vi "parking_ung2rev.vi"() -> ()   [LabVIEW 2012]
uses:
  G_SEN.vi
  G_NAV.vi
  G_VEH.vi
  G_PATH.vi
panel:
  out "M6006":T1={"GPSTime"=22892800.0, "attitude[2]"=-0.6123908, "lcc[0]"=-970.47205, "lcc[1]"=200.52362, "heading_GPS"=-0.6106907} {"GPSTime" format="%#_6f"}
  in  "a":dbl=0.1
  out "parkingpoint":dbl[][](array[numeric])=[[461.5244031818319, -787.8333505670688, 1.0792755610756257], [466.2440748318668, -779.0171892983614, 1.0792755610756257], [467.4239927443755, -776.8131489811844, 1.0792755610756257], [468.60391065688424, -774.6091086640076, 0.48978457392345476], [475.6187081476555, -773.2417442369818, -0.09970641322871643], [485.5690424693232, -774.2371571598643, -0.09970641322871643]]
  out "size":i32=12
  out "sizex":i32=12
  out "sizey":i32=1
  out "xmin":dbl=-1.5
  out "mapzero":dbl[][](array[numeric])
  out "XY Graph":cluster{"Y":dbl[], "Y":dbl[]}[](graph)=[{"Y"=[], "Y"=[]}, {"Y"=[], "Y"=[]}, {"Y"=[], "Y"=[]}, {"Y"=array[1422 elements], "Y"=array[1422 elements]}, {"Y"=[], "Y"=[]}, {"Y"=[0.5023373790116399, 1.0005000639291148, -1.499467549798603, -1.9976302347160777, 0.5023373790116399], "Y"=[3.2753448651924955, -1.6997766347666685, -1.950100285891864, 3.0250212140673, 3.2753448651924955]}]
  out "time":u32
  out "box":dbl[][](array[numeric])
  out "lane":dbl[][](array[numeric])
  out "obs":dbl[][](array[numeric])
  out "y_min":dbl=-2.25
  out "tic":u32=336134883
  out "sensor_lane":dbl[][](array[numeric])
  out "sensor_obs":dbl[][](array[numeric])
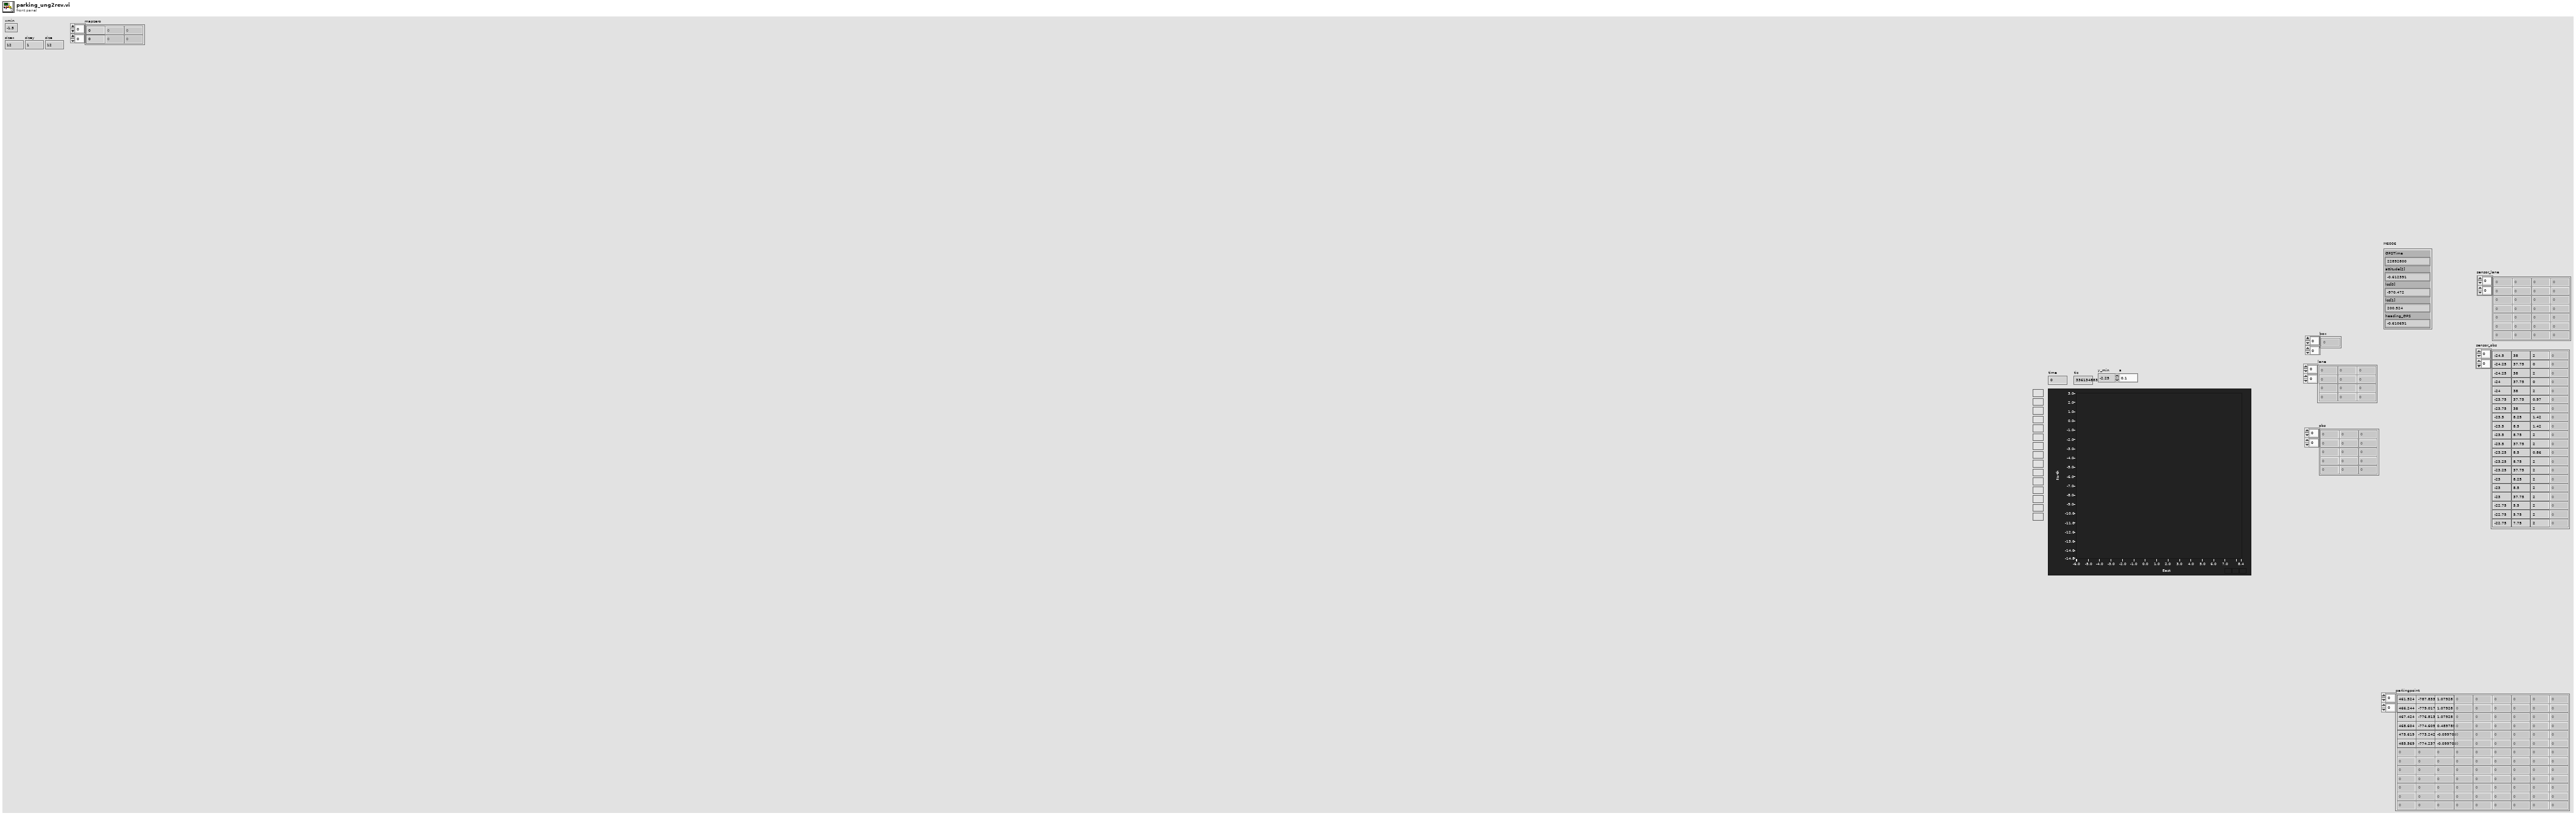
[diagram p1: front panel]
types:
  T1 = cluster{"GPSTime":dbl, "attitude[2]":sgl, "lcc[0]":sgl, "lcc[1]":sgl, "heading_GPS":sgl}
  T2 = cluster{"GPSTime":dbl, "attitude[2]":dbl, "lcc[0]":dbl, "lcc[1]":dbl, "heading_GPS":dbl}
  T3 = cluster{"idx":i32, "x":dbl, "y":dbl, "h":dbl, "x_path":dbl}
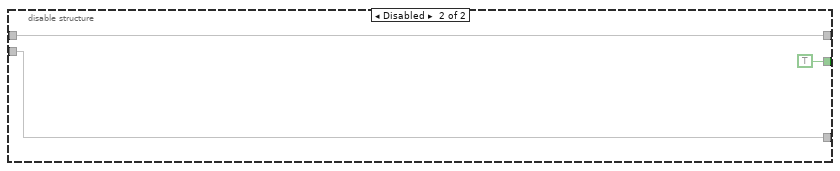
[diagram p3: hidden frame]
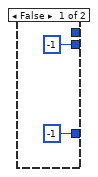
[diagram p6: hidden frame]
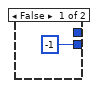
[diagram p7: hidden frame]
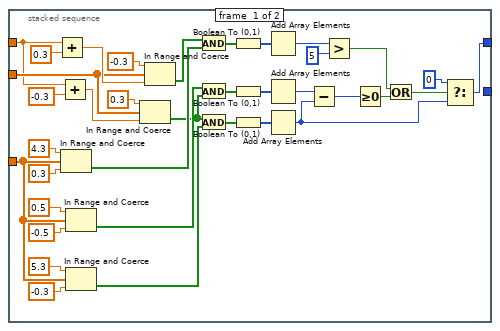
[diagram p8: hidden frame]
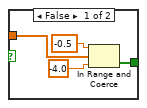
[diagram p10: hidden frame]
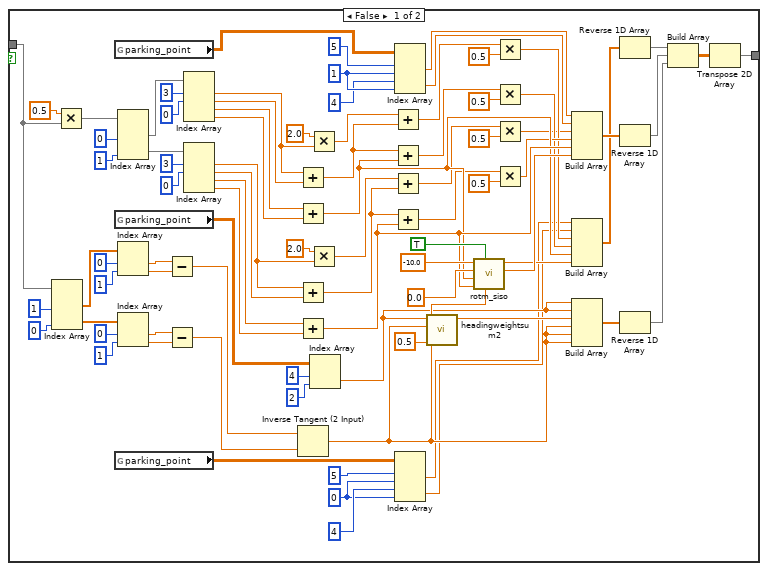
[diagram p13: hidden frame]
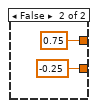
[diagram p16: hidden frame]
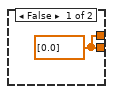
[diagram p17: hidden frame]
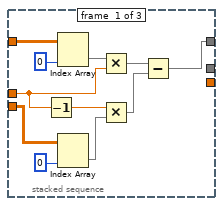
[diagram p18: hidden frame]
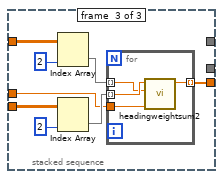
[diagram p19: hidden frame]
diagram:
  n1 = flat-sequence {
    tunnel: [w865] -> w2
    tunnel: [w864] -> w1
    tunnel: w2 -> [w878]
    tunnel: w1 -> [w877]
    frame #0 {
      n2 = disable-structure shown="Disabled" {
        disable-tunnel: [w10 _] -> w7
        frame Disabled {
          n3 = local read "sensor_obs"() -> (w10:dbl[][])
        }
        frame Enabled {
        }
      }
      "obs" <- w7
      n4 = Tick Count (ms)() -> (millisecond timer value=→"tic":u32)
      n5 = global read "G_SEN.vi" "sensor_lane"() -> (w6:dbl[][])
      n6 = global read "G_SEN.vi" "sensor_obs"() -> (→"sensor_obs":dbl[][])
      n7 = global read "G_SEN.vi" "sensor_etc"() -> (w5:dbl[][])
      n8 = global read "G_NAV.vi" "M6006"() -> (→"M6006":T2)
      n9 = Build Array (concatenate)(w5, w6) -> (→"sensor_lane":dbl[][])
    }
    frame #1 {
      n10 = local read "sensor_lane"() -> (w17:dbl[][])
      n11 = Index Array(array=w17, index (col) #1=0 ("disabled index (col)")) -> (element #1=w15:dbl[], element #2=w14:dbl[])  [unwired: 3 in]
      n12 = disable-structure shown="Enabled" {
        disable-tunnel: w15 -> [w31 w57]
        disable-tunnel: w14 -> [w30 w56]
        disable-tunnel: [w21 w56] -> w13
        disable-tunnel: [w22 w57] -> w12
        disable-tunnel: [w26 TRUE] -> w11
        frame Enabled {
          n13 = local read "M6006"() -> (w47:T1)
          n14 = Unbundle By Name(w47) -> ("lcc[1]"=w44:sgl, "lcc[0]"=w45:sgl, "attitude[2]"=w46:sgl)
          n15 = global read "G_VEH.vi" "xparking"() -> (w50:T3)
          n16 = Negate(x=w46) -> (-x=w43:sgl)
          n17 = Unbundle By Name(w50) -> ("x"=w49:dbl, "y"=w48:dbl)
          n18 = call "rotm_siso.vi"("angle[rad]"=w43, "y0"=w45, "x0"=w44, "y"=w48, "x"=w49) -> ("y'"=w41:dbl, "x'"=w42:dbl)  [unwired: 5 in]
          n19 = Subtract(x=w31, y=w42) -> (x-y=w39:dbl[])
          n20 = Subtract(x=w30, y=w41) -> (x-y=w40:dbl[])
          n21 = Square(x=w39) -> (x^2=w38:dbl[])
          n22 = Square(x=w40) -> (x^2=w37:dbl[])
          n23 = Add(x=w38, y=w37) -> (x+y=w36:dbl[])
          n24 = Square Root(x=w36) -> (sqrt(x)=w35:dbl[])
          n25 = Less Or Equal?(x=w35, y=3.0) -> (x <= y?=w33:bool[])
          n26 = Boolean To (0,1)(Boolean=w33) -> (0, 1=w32:i16[])
          n27 = Build Cluster Array(w32, w31, w30) -> (w29:cluster{i16, "element":dbl, "element":dbl}[])
          n28 = Sort 1D Array(array=w29) -> (sorted array=w28:cluster{i16, "element":dbl, "element":dbl}[])
          n29 = for {
            tunnel: w28 -> [w54] mode=indexing
            tunnel: [w53] -> w25 mode=indexing
            tunnel: [w52] -> w24 mode=indexing
            tunnel: [w51] -> w23 mode=indexing
            n30 = Unbundle(w54) -> (w51:i16, "element"=w53:dbl, "element"=w52:dbl)
          }
          n31 = Add Array Elements(numeric array=w23) -> (sum=w19:i16)
          n32 = Array Max & Min(array=w23) -> (max value=w27:i16, max index (indices)=w20:i32)  [unwired: 2 out]
          n33 = Not Equal To 0?(x=w27) -> (x != 0?=w26:bool)
          n34 = Array Subset(array=w25, index=w20, length=w19) -> (w22:dbl[])
          n35 = Array Subset(array=w24, index=w20, length=w19) -> (w21:dbl[])
        }
        frame Disabled {
        }
      }
      n36 = case shown="True" w11 {
        tunnel: w13 -> [_ w58]
        tunnel: w12 -> [_ w60]
        tunnel: [_ w66] -> w18
        frame False {
        }
        frame True {
          n37 = Array Max & Min(array=w60) -> (max value=w65:dbl, min value=w64:dbl)  [unwired: 2 out]
          n38 = Array Max & Min(array=w58) -> (max value=w63:dbl, min value=w62:dbl)  [unwired: 2 out]
          n39 = flat-sequence {
            tunnel: w65 -> [w79]
            tunnel: w64 -> [w78]
            tunnel: w63 -> [w77]
            tunnel: w62 -> [w76]
            tunnel: [w69] -> w61
            tunnel: w60 -> [w69]
            tunnel: [w68] -> w59
            tunnel: w58 -> [w68]
            tunnel: [w117] -> w67
            tunnel: w61 -> [w106]
            tunnel: w59 -> [w105]
            tunnel: w67 -> [w148]
            tunnel: [w147] -> w66
            frame #0 {
              n40 = flat-sequence {
                tunnel: w79 -> [w83]
                tunnel: w78 -> [w82]
                tunnel: w77 -> [_]
                tunnel: w76 -> [w81]
                tunnel: [w83] -> w75
                tunnel: [w82] -> w74
                tunnel: [0.0] -> w73
                tunnel: [w81] -> w72
                tunnel: w75 -> [w100]
                tunnel: w74 -> [w99]
                tunnel: w73 -> [w94]
                tunnel: w72 -> [w93]
                tunnel: [w91] -> w71
                tunnel: [w90] -> w70
                tunnel: w71 -> [w103]
                tunnel: w70 -> [w102]
                frame #0 {
                  "y_min" <- w81
                  "xmin" <- w82
                }
                frame #1 {
                  n41 = Subtract(x=w100, y=w99) -> (x-y=w98:dbl)
                  n42 = Subtract(x=w94, y=w93) -> (x-y=w95:dbl)
                  n43 = Multiply(x=w98, y=4.0) -> (x*y=w89:dbl)
                  n44 = Multiply(x=w95, y=4.0) -> (x*y=w88:dbl)
                  n45 = Round Toward +Infinity(x=w89) -> (ceil(x): smallest int >= x=w84:dbl)
                  n46 = Round Toward +Infinity(x=w88) -> (ceil(x): smallest int >= x=w87:dbl)
                  n47 = Increment(x=w84) -> (x+1=w85:dbl)
                  n48 = Increment(x=w87) -> (x+1=w86:dbl)
                  n49 = To Long Integer(number=w85) -> (32bit integer=w91:i32)
                  "sizex" <- w91
                  n50 = To Long Integer(number=w86) -> (32bit integer=w90:i32)
                  "sizey" <- w90
                  n51 = Multiply(x=w91, y=w90) -> (x*y=→"size":i32)
                }
                frame #2 {
                  n52 = Initialize Array(0.0, w103, w102) -> (→"mapzero":dbl[][])
                }
              }
            }
            frame #1 {
              n53 = local read "y_min"() -> (w111:dbl)
              n54 = local read "xmin"() -> (w108:dbl)
              n55 = local read "mapzero"() -> (w107:dbl[][])
              n56 = Subtract(x=w106, y=w108) -> (x-y=w116:dbl[])
              n57 = Subtract(x=w105, y=w111) -> (x-y=w110:dbl[])
              n58 = Multiply(x=w116, y=4.0) -> (x*y=w114:dbl[])
              n59 = Multiply(x=4.0, y=w110) -> (x*y=w115:dbl[])
              n60 = To Long Integer(number=w114) -> (32bit integer=w113:i32[])
              n61 = To Long Integer(number=w115) -> (32bit integer=w112:i32[])
              n62 = for {
                tunnel: w113 -> [w123] mode=indexing
                shift-right: [w122] -> w117
                shift-left: w107 -> [w120]
                tunnel: w112 -> [w121] mode=indexing
                n63 = Replace Array Subset(array=w120, new element=1.0 ("new element/subarray"), index (row)=w123, index (col)=w121) -> (w122:dbl[][])
              }
            }
            frame #2 {
              n64 = local read "sizey"() -> (w138:i32)
              n65 = local read "sizex"() -> (w143:i32)
              n66 = local read "size"() -> (w124:i32)
              n67 = for {
                N: w138 -> [_]
                tunnel: [w168] -> w137 mode=indexing
                i -> [w168]
              }
              n68 = Reshape Array(w148, w124) -> (w144:dbl[])
              n69 = for {
                N: w143 -> [_]
                tunnel: [w169] -> w142 mode=concatenating
                i -> [w171]
                n70 = local read "sizey"() -> (w170:i32)
                n71 = Initialize Array(w171, w170) -> (w169:i32[])
              }
              n72 = Not Equal To 0?(x=w144) -> (x != 0?=w126:bool[])
              n73 = Boolean To (0,1)(Boolean=w126) -> (0, 1=w131:i16[])
              n74 = Add Array Elements(numeric array=w131) -> (sum=w129:i16)
              n75 = Multiply(x=w137, y=0.25) -> (x*y=w134:dbl[])
              n76 = local read "y_min"() -> (w135:dbl)
              n77 = Multiply(x=w142, y=0.25) -> (x*y=w139:dbl[])
              n78 = local read "xmin"() -> (w140:dbl)
              n79 = Add(x=w134, y=w135) -> (x+y=w132:dbl[])
              n80 = local read "sizex"() -> (w133:i32)
              n81 = Add(x=w139, y=w140) -> (x+y=w146:dbl[])
              n82 = for {
                N: w133 -> [_]
                tunnel: w132 -> [w167]
                tunnel: [w167] -> w145 mode=concatenating
              }
              n83 = Initialize Array(0.0 ("element"), w129, 3 ("dimension size")) -> (w127:dbl[][])
              n84 = for {
                tunnel: w145 -> [w156] mode=indexing
                tunnel: w146 -> [w155] mode=indexing
                tunnel: w144 -> [w152] mode=indexing
                shift-right: [w153] -> w147
                shift-left: w127 -> [w154]
                tunnel: w126 -> [w151] mode=indexing
                shift-right: [w149] -> _
                shift-left: 0 -> [w150]
                n85 = case shown="True" w151 {
                  tunnel: w156 -> [_ w165]
                  tunnel: w155 -> [_ w166]
                  tunnel: w152 -> [_ w164]
                  tunnel: w154 -> [w158 w163]
                  tunnel: [w158 w162] -> w153
                  tunnel: w150 -> [w157 w160]
                  tunnel: [w157 w159] -> w149
                  frame False {
                  }
                  frame True {
                    n86 = Build Array(w166, w165, w164) -> (w161:dbl[])
                    n87 = Increment(x=w160) -> (x+1=w159:i32)
                    n88 = Replace Array Subset(array=w163, new element=w161, index (row)=w160) -> (w162:dbl[][])  [unwired: 1 in]
                  }
                }
              }
            }
          }
        }
      }
      "lane" <- w18
    }
    frame #2 {
      n89 = flat-sequence {
        tunnel: [w173] -> w172
        frame #0 {
          n90 = flat-sequence {
            tunnel: [w181] -> w176
            tunnel: [w179] -> w175
            tunnel: [w180] -> w174
            tunnel: w176 -> [w318]
            tunnel: w175 -> [w324]
            tunnel: w174 -> [w319]
            tunnel: [w316] -> w173
            frame #0 {
              n91 = local read "lane"() -> (w183:dbl[][])
              n92 = Index Array(array=w183, index (col) #1=1 ("disabled index (col)"), index (col) #2=0 ("index (col)")) -> (element #1=w178:dbl[], element #2=w177:dbl[])  [unwired: 2 in]
              n93 = for {
                tunnel: w177 -> [w192]
                tunnel: w178 -> [w193]
                tunnel: [w198] -> w181 mode=indexing
                tunnel: [w197] -> w180 mode=indexing
                tunnel: [w196] -> w179 mode=indexing
                tunnel: w178 -> [w191] mode=indexing
                tunnel: w177 -> [w190] mode=indexing
                n94 = Subtract(x=w193, y=w191) -> (x-y=w202:dbl[])
                n95 = Subtract(x=w192, y=w190) -> (x-y=w201:dbl[])
                n96 = global read "G_PATH.vi" "parking_width"() -> (w185:dbl)
                n97 = Square(x=w202) -> (x^2=w205:dbl[])
                n98 = Square(x=w201) -> (x^2=w204:dbl[])
                n99 = Inverse Tangent (2 Input)(1:w201, 2:w202) -> (0:w195:dbl[])
                n100 = Add(x=w205, y=w204) -> (x+y=w200:dbl[])
                n101 = Square Root(x=w200) -> (sqrt(x)=w199:dbl[])
                n102 = Add(x=0.6, y=w185) -> (x+y=w186:dbl)
                n103 = Subtract(x=w185, y=0.6) -> (x-y=w188:dbl)
                n104 = In Range and Coerce(upper limit=w186, x=w199, lower limit=w188) -> (In Range?=w194:bool[])  [unwired: 1 out]
                n105 = Or Array Elements(Boolean array=w194) -> (logical OR=w203:bool)
                n106 = case shown="True" w203 {
                  tunnel: w194 -> [_ w220]
                  tunnel: w202 -> [_ w219]
                  tunnel: w201 -> [_ w218]
                  tunnel: w195 -> [_ w217]
                  tunnel: w199 -> [_ w210]
                  tunnel: [_ w212] -> w198
                  tunnel: [-1 ("element") w216] -> w197
                  tunnel: [-1 ("element") w213] -> w196
                  frame False {
                  }
                  frame True {
                    n107 = Negate(x=w210) -> (-x=w209:dbl[])
                    n108 = for {
                      tunnel: w220 -> [w228] mode=indexing
                      tunnel: w219 -> [w227]
                      tunnel: w218 -> [w226]
                      tunnel: w217 -> [w225] mode=indexing
                      tunnel: w209 -> [w224] mode=indexing
                      tunnel: [w223] -> w215 mode=indexing
                      tunnel: [w222] -> w214 mode=indexing
                      tunnel: [w221] -> w208 mode=indexing
                      i -> [w222]
                      n109 = case shown="True" w228 {
                        tunnel: w227 -> [_ w242]
                        tunnel: w226 -> [_ w241]
                        tunnel: w225 -> [_ w239]
                        tunnel: w224 -> [_ w235]
                        tunnel: [-1 w230] -> w223
                        tunnel: [_ w231] -> w221
                        frame False {
                        }
                        frame True {
                          w240 = 0.0 ("y0")
                          n110 = call "rotm_mimo.vi"("angle[rad]"=w239, "y0"=w240, "x0"=w240, "y"=w242, "x"=w241) -> ("Y"=w237:dbl[], "X"=w238:dbl[])  [unwired: 3 in, 2 out]
                          n111 = Negate(x=w238) -> (-x=w236:dbl[])
                          n112 = stacked-sequence {
                            tunnel: w237 -> [w256 w293]
                            tunnel: w236 -> [w261 w297]
                            tunnel: w235 -> [w260 w296]
                            tunnel: [w259 _] -> w234
                            tunnel: [_ w283] -> w233
                            frame #0 {
                              n113 = Add(x=w260, y=0.3) -> (x+y=w266:dbl)
                              n114 = Add(x=w260, y=-0.3) -> (x+y=w274:dbl)
                              n115 = In Range and Coerce(upper limit=4.3, x=w256, lower limit=0.3) -> (In Range?=w268:bool[])  [unwired: 1 out]
                              n116 = In Range and Coerce(upper limit=0.5, x=w256, lower limit=-0.5) -> (In Range?=w255:bool[])  [unwired: 1 out]
                              n117 = In Range and Coerce(upper limit=5.3, x=w256, lower limit=-0.3) -> (In Range?=w273:bool[])  [unwired: 1 out]
                              n118 = In Range and Coerce(upper limit=0.3, x=w261, lower limit=w274) -> (In Range?=w254:bool[])  [unwired: 1 out]
                              n119 = In Range and Coerce(upper limit=-0.3, x=w261, lower limit=w266) -> (In Range?=w267:bool[])  [unwired: 1 out]
                              n120 = And(x=w267, y=w268) -> (x .and. y?=w269:bool[])
                              n121 = And(x=w255, y=w254) -> (x .and. y?=w252:bool[])
                              n122 = And(x=w254, y=w273) -> (x .and. y?=w272:bool[])
                              n123 = Boolean To (0,1)(Boolean=w269) -> (0, 1=w270:i16[])
                              n124 = Boolean To (0,1)(Boolean=w252) -> (0, 1=w253:i16[])
                              n125 = Boolean To (0,1)(Boolean=w272) -> (0, 1=w271:i16[])
                              n126 = Add Array Elements(numeric array=w270) -> (sum=w246:i16)
                              n127 = Add Array Elements(numeric array=w253) -> (sum=w251:i16)
                              n128 = Add Array Elements(numeric array=w271) -> (sum=w244:i16)
                              n129 = Subtract(x=w251, y=w244) -> (x-y=w250:i16)
                              n130 = Greater?(x=w246, y=i16 5) -> (0:w249:bool)
                              n131 = Greater Or Equal To 0?(x=w250) -> (x >= 0?=w248:bool)
                              n132 = Or(x=w249, y=w248) -> (x .or. y?=w247:bool)
                              n133 = Select(t=i16 0, s=w247, f=w244) -> (s? t:f=w259:i16)
                            }
                            frame #1 {
                              n134 = Add(x=w296, y=0.3) -> (x+y=w302:dbl)
                              n135 = Add(x=w296, y=-0.3) -> (x+y=w310:dbl)
                              n136 = In Range and Coerce(upper limit=-0.3, x=w293, lower limit=-4.3) -> (In Range?=w304:bool[])  [unwired: 1 out]
                              n137 = In Range and Coerce(upper limit=0.5, x=w293, lower limit=-0.5) -> (In Range?=w292:bool[])  [unwired: 1 out]
                              n138 = In Range and Coerce(upper limit=0.3, x=w293, lower limit=-5.3) -> (In Range?=w309:bool[])  [unwired: 1 out]
                              n139 = In Range and Coerce(upper limit=0.3, x=w297, lower limit=w310) -> (In Range?=w291:bool[])  [unwired: 1 out]
                              n140 = In Range and Coerce(upper limit=-0.3, x=w297, lower limit=w302) -> (In Range?=w303:bool[])  [unwired: 1 out]
                              n141 = And(x=w303, y=w304) -> (x .and. y?=w305:bool[])
                              n142 = And(x=w292, y=w291) -> (x .and. y?=w289:bool[])
                              n143 = And(x=w291, y=w309) -> (x .and. y?=w308:bool[])
                              n144 = Boolean To (0,1)(Boolean=w305) -> (0, 1=w306:i16[])
                              n145 = Boolean To (0,1)(Boolean=w289) -> (0, 1=w290:i16[])
                              n146 = Boolean To (0,1)(Boolean=w308) -> (0, 1=w307:i16[])
                              n147 = Add Array Elements(numeric array=w306) -> (sum=w282:i16)
                              n148 = Add Array Elements(numeric array=w290) -> (sum=w288:i16)
                              n149 = Add Array Elements(numeric array=w307) -> (sum=w280:i16)
                              n150 = Subtract(x=w288, y=w280) -> (x-y=w287:i16)
                              n151 = Greater?(x=w282, y=i16 5) -> (0:w286:bool)
                              n152 = Greater Or Equal To 0?(x=w287) -> (x >= 0?=w285:bool)
                              n153 = Or(x=w286, y=w285) -> (x .or. y?=w284:bool)
                              n154 = Select(t=i16 0, s=w284, f=w280) -> (s? t:f=w283:i16)
                            }
                          }
                          n155 = Build Array(w234, w233) -> (w232:i16[])
                          n156 = Array Max & Min(array=w232) -> (max value=w231:i16, max index (indices)=w230:i32)  [unwired: 2 out]
                        }
                      }
                    }
                    n157 = Array Max & Min(array=w208) -> (max value=w212:i16, max index (indices)=w211:i32)  [unwired: 2 out]
                    n158 = Index Array(array=w214, index=w211) -> (element=w213:i32)
                    n159 = Index Array(array=w215, index=w211) -> (element=w216:i32)
                  }
                }
              }
            }
            frame #1 {
              n160 = Array Max & Min(array=w318) -> (max value=w320:i16, max index (indices)=w315:i32)  [unwired: 2 out]
              n161 = Index Array(array=w324, index=w315) -> (element=w321:i32)
              n162 = Index Array(array=w319, index=w315) -> (element=w322:i32)
              n163 = Greater Or Equal?(x=w320, y=i16 4) -> (x >= y?=w317:bool)
              n164 = case shown="True" w317 {
                tunnel: w321 -> [_ w364]
                tunnel: w322 -> [_ w342]
                tunnel: [_ w341] -> w316
                tunnel: w315 -> [_ w325]
                frame False {
                }
                frame True {
                  w347 = 0.0 ("element")
                  w344 = dbl[] [0.0, 5.0, 5.0, 0.0]
                  n165 = local read "lane"() -> (w365:dbl[][])
                  n166 = Negate(x=w344) -> (-x=w343:dbl[])
                  n167 = Index Array(array=w365, index (row) #1=w364, index (row) #2=w325) -> (element #1=w363:dbl[], element #2=w357:dbl[])  [unwired: 2 in]
                  n168 = Equal To 0?(x=w342) -> (x = 0?=w326:bool)
                  n169 = Subtract(x=w363, y=w357) -> (x-y=w351:dbl[])
                  n170 = Select(t=w344, s=w326, f=w343) -> (s? t:f=w345:dbl[])
                  n171 = Square(x=w351) -> (x^2=w350:dbl[])
                  n172 = Index Array(array=w351, index #1=1 ("index"), index #2=0 ("index")) -> (element #1=w360:dbl, element #2=w359:dbl)
                  n173 = Add Array Elements(numeric array=w350) -> (sum=w349:dbl)
                  n174 = Inverse Tangent (2 Input)(1:w359, 2:w360) -> (0:w353:dbl)
                  n175 = Square Root(x=w349) -> (sqrt(x)=w348:dbl)
                  n176 = call "headingoperater.vi"("h1"=w353, "h2"=1.5707963267948966) -> ("h2+h1"=w331:dbl)  [unwired: 8 in, 1 out]
                  n177 = Negate(x=w348) -> (-x=w327:dbl)
                  n178 = Index Array(array=w357, index #1=0 ("index")) -> (element #1=w333:dbl, element #2=w332:dbl)  [unwired: 1 in]
                  n179 = flat-sequence {
                    tunnel: [w371] -> w330
                    tunnel: w333 -> [w370]
                    tunnel: w332 -> [w369]
                    tunnel: w331 -> [w368]
                    tunnel: w327 -> [w367]
                    tunnel: w326 -> [w366]
                    frame #0 {
                      n180 = disable-structure shown="Enabled" {
                        disable-tunnel: [w379 _] -> w371
                        disable-tunnel: w370 -> [w378 _]
                        disable-tunnel: w369 -> [w377 _]
                        disable-tunnel: w368 -> [w376 _]
                        disable-tunnel: w367 -> [w375 _]
                        disable-tunnel: w366 -> [w374 _]
                        frame Enabled {
                          n181 = local read "sensor_obs"() -> (w391:dbl[][])
                          n182 = Index Array(array=w391, index (col) #1=0 ("disabled index (col)"), index (col) #2=1 ("index (col)")) -> (element #1=w388:dbl[], element #2=w387:dbl[])  [unwired: 2 in]
                          n183 = call "rotm_mimo.vi"("angle[rad]"=w376, "reverse"=FALSE, "y0"=w377, "x0"=w378, "y"=w387, "x"=w388) -> ("Y"=w383:dbl[], "X"=w385:dbl[])  [unwired: 2 in, 2 out]
                          n184 = Add(x=0.2, y=w375) -> (x+y=w381:dbl)
                          n185 = case shown="True" w374 {
                            tunnel: w385 -> [w394 w399]
                            tunnel: [w392 w396] -> w373
                            frame False {
                              n186 = In Range and Coerce(upper limit=-0.5, x=w394, lower limit=-4.0) -> (In Range?=w392:bool[])  [unwired: 1 out]
                            }
                            frame True {
                              n187 = In Range and Coerce(upper limit=4.0, x=w399, lower limit=0.5) -> (In Range?=w396:bool[])  [unwired: 1 out]
                            }
                          }
                          n188 = In Range and Coerce(upper limit=-0.2, x=w383, lower limit=w381) -> (In Range?=w372:bool[])  [unwired: 1 out]
                          n189 = And(x=w372, y=w373) -> (x .and. y?=w380:bool[])
                          n190 = Or Array Elements(Boolean array=w380) -> (logical OR=w379:bool)
                        }
                        frame Disabled {
                        }
                      }
                    }
                  }
                  n191 = Build Array(w347, w347, w327, w327) -> (w346:dbl[])
                  n192 = call "rotm_mimo.vi"("angle[rad]"=w331, "reverse"=TRUE, "y0"=w332, "x0"=w333, "y"=w346, "x"=w345) -> ("Y"=w355:dbl[], "X"=w338:dbl[])  [unwired: 2 in, 2 out]
                  n193 = Add Array Elements(numeric array=w338) -> (sum=w337:dbl)
                  n194 = Build Array(w338, w355) -> (w354:dbl[][])
                  n195 = Transpose 2D Array(2D array=w354) -> (transposed array=w340:dbl[][])
                  n196 = Multiply(x=0.25, y=w337) -> (x*y=w335:dbl)
                  n197 = Greater?(x=w335, y=7.0) -> (0:w329:bool)
                  n198 = Or(x=w330, y=w329) -> (x .or. y?=w328:bool)
                  n199 = Select(t=dbl[][] [], s=w328, f=w340) -> (s? t:f=w341:dbl[][])
                }
              }
            }
          }
        }
      }
      "box" <- w172
    }
    frame #3 {
      n200 = local read "box"() -> (w401:dbl[][])
      n201 = Empty Array?(array=w401) -> (empty?=w400:bool)
      n202 = case shown="False" w400 {
        frame False {
          n203 = flat-sequence {
            tunnel: [w406] -> w402
            tunnel: w402 -> [w488]
            frame #0 {
              n204 = local read "M6006"() -> (w444:T1)
              n205 = local read "box"() -> (w409:dbl[][])
              n206 = Unbundle By Name(w444) -> ("lcc[1]"=w440:sgl, "lcc[0]"=w439:sgl, "attitude[2]"=w443:sgl)
              n207 = Array Subset(array=w409, length (row)=4 ("length")) -> (w408:dbl[][])  [unwired: 3 in]
              n208 = Negate(x=w443) -> (-x=w442:sgl)
              n209 = Index Array(array=w408, index (col) #1=0 ("disabled index (col)")) -> (element #1=w446:dbl[], element #2=w445:dbl[])  [unwired: 3 in]
              n210 = call "rotm_mimo.vi"("angle[rad]"=w442, "reverse"=TRUE, "y0"=w439, "x0"=w440, "y"=w445, "x"=w446) -> ("Y"=w431:dbl[], "X"=w433:dbl[])  [unwired: 2 in, 2 out]
              n211 = Subtract(x=w433, y=w440) -> (x-y=w437:dbl[])
              n212 = Subtract(x=w431, y=w439) -> (x-y=w438:dbl[])
              n213 = Square(x=w437) -> (x^2=w436:dbl[])
              n214 = Square(x=w438) -> (x^2=w435:dbl[])
              n215 = Add(x=w436, y=w435) -> (x+y=w434:dbl[])
              n216 = Array Max & Min(array=w434) -> (min index (indices)=w432:i32)  [unwired: 3 out]
              n217 = Delete From Array(array=w433, index=w432) -> (deleted portion=w419:dbl, array with subset deleted=w423:dbl[])  [unwired: 1 in]
              n218 = Delete From Array(array=w431, index=w432) -> (deleted portion=w403:dbl, array with subset deleted=w415:dbl[])  [unwired: 1 in]
              n219 = Subtract(x=w423, y=w419) -> (x-y=w427:dbl[])
              n220 = Subtract(x=w415, y=w403) -> (x-y=w426:dbl[])
              n221 = Square(x=w427) -> (x^2=w428:dbl[])
              n222 = Square(x=w426) -> (x^2=w429:dbl[])
              n223 = Add(x=w428, y=w429) -> (x+y=w430:dbl[])
              n224 = Array Max & Min(array=w430) -> (max index (indices)=w413:i32, min index (indices)=w412:i32)  [unwired: 2 out]
              n225 = Add(x=w413, y=w412) -> (x+y=w425:i32)
              n226 = Subtract(x=3, y=w425) -> (x-y=w414:i32)
              n227 = Index Array(array=w423, index #1=w414, index #2=w413, index #3=w412) -> (element #1=w422:dbl, element #2=w421:dbl, element #3=w420:dbl)
              n228 = Index Array(array=w415, index #1=w414, index #2=w413, index #3=w412) -> (element #1=w416:dbl, element #2=w417:dbl, element #3=w418:dbl)
              n229 = Build Array(w419, w422, w421, w420) -> (w411:dbl[])
              n230 = Build Array(w403, w416, w417, w418) -> (w410:dbl[])
              n231 = flat-sequence {
                tunnel: w410 -> [w448]
                tunnel: w411 -> [w451]
                tunnel: [w450] -> w405
                tunnel: [w449] -> w404
                tunnel: [w483] -> w406
                tunnel: w405 -> [w486]
                tunnel: w404 -> [w485]
                frame #0 {
                  n232 = Index Array(array=w451, index #1=1 ("index"), index #2=0 ("index"), index #3=2 ("index"), index #4=1 ("index")) -> (element #1=w469:dbl, element #2=w470:dbl, element #3=w464:dbl, element #4=w463:dbl)
                  n233 = Index Array(array=w448, index #1=2 ("index"), index #2=1 ("index"), index #3=1 ("index"), index #4=0 ("index")) -> (element #1=w472:dbl, element #2=w471:dbl, element #3=w460:dbl, element #4=w459:dbl)
                  n234 = Subtract(x=w469, y=w470) -> (x-y=w468:dbl)
                  n235 = Subtract(x=w464, y=w463) -> (x-y=w457:dbl)
                  n236 = Subtract(x=w472, y=w471) -> (x-y=w467:dbl)
                  n237 = Subtract(x=w460, y=w459) -> (x-y=w458:dbl)
                  n238 = Multiply(x=w468, y=w467) -> (x*y=w456:dbl)
                  n239 = Multiply(x=w457, y=w458) -> (x*y=w455:dbl)
                  n240 = Subtract(x=w456, y=w455) -> (x-y=w454:dbl)
                  n241 = Sign(1:w454) -> (0:w453:dbl)
                  n242 = Greater Than 0?(x=w453) -> (x > 0?=w452:bool)
                  n243 = case shown="False" w452 {
                    tunnel: w451 -> [w480 w482]
                    tunnel: [w479 w482] -> w450
                    tunnel: [w477 w481] -> w449
                    tunnel: w448 -> [w478 w481]
                    frame False {
                      n244 = Reverse 1D Array(array=w480) -> (reversed array=w479:dbl[])
                      n245 = Reverse 1D Array(array=w478) -> (reversed array=w477:dbl[])
                    }
                    frame True {
                    }
                  }
                }
                frame #1 {
                  n246 = Build Array(w486, w485) -> (w484:dbl[][])
                  n247 = Transpose 2D Array(2D array=w484) -> (transposed array=w483:dbl[][])
                }
              }
            }
            frame #1 {
              n248 = global read "G_VEH.vi" "parking_loop"() -> (w487:bool)
              n249 = case shown="True" w487 {
                tunnel: [w560 w635] -> w489
                tunnel: w488 -> [w514 w589]
                frame False {
                  w517 = 1 ("disabled index (col)")
                  w518 = 0 ("disabled index (col)")
                  n250 = Index Array(array=w514, index (col) #1=1 ("disabled index (col)"), index (col) #2=0 ("index (col)")) -> (element #1=w558:dbl[], element #2=w553:dbl[])  [unwired: 2 in]
                  n251 = Multiply(x=0.5, y=w514) -> (x*y=w531:dbl[][])
                  n252 = global read "G_PATH.vi" "parking_point"() -> (w490:dbl[][])
                  n253 = global read "G_PATH.vi" "parking_point"() -> (w491:dbl[][])
                  n254 = global read "G_PATH.vi" "parking_point"() -> (w492:dbl[][])
                  n255 = Index Array(array=w531, index (col) #1=0 ("disabled index (col)"), index (col) #2=1 ("index (col)")) -> (element #1=w525:dbl[], element #2=w544:dbl[])  [unwired: 2 in]
                  n256 = Index Array(array=w558, index #1=0 ("index"), index #2=1 ("index")) -> (element #1=w550:dbl, element #2=w549:dbl)
                  n257 = Index Array(array=w553, index #1=0 ("index"), index #2=1 ("index")) -> (element #1=w548:dbl, element #2=w547:dbl)
                  n258 = Subtract(x=w550, y=w549) -> (x-y=w546:dbl)
                  n259 = Subtract(x=w548, y=w547) -> (x-y=w545:dbl)
                  n260 = Index Array(array=w525, index #1=3 ("index"), index #2=0 ("index")) -> (element #1=w513:dbl, element #2=w528:dbl, element #3=w529:dbl, element #4=w530:dbl)  [unwired: 2 in]
                  n261 = Index Array(array=w544, index #1=3 ("index"), index #2=0 ("index")) -> (element #1=w511:dbl, element #2=w541:dbl, element #3=w540:dbl, element #4=w539:dbl)  [unwired: 2 in]
                  n262 = Add(x=w513, y=w528) -> (x+y=w508:dbl)
                  n263 = Add(x=w529, y=w530) -> (x+y=w568:dbl)
                  n264 = Add(x=w511, y=w541) -> (x+y=w503:dbl)
                  n265 = Add(x=w540, y=w539) -> (x+y=w569:dbl)
                  n266 = Inverse Tangent (2 Input)(1:w545, 2:w546) -> (0:w509:dbl)
                  n267 = Multiply(x=2.0, y=w513) -> (x*y=w507:dbl)
                  n268 = Multiply(x=2.0, y=w511) -> (x*y=w502:dbl)
                  n269 = Index Array(array=w491, index (row)=4, index (col)=2 ("disabled index (col)")) -> (element=w497:dbl)
                  n270 = Add(x=w507, y=w508) -> (x+y=w505:dbl)
                  n271 = Add(x=w508, y=w568) -> (x+y=w533:dbl)
                  n272 = Add(x=w502, y=w503) -> (x+y=w500:dbl)
                  n273 = Add(x=w503, y=w569) -> (x+y=w538:dbl)
                  n274 = Index Array(array=w490, index (row) #1=5 ("index (row)"), index (col) #1=w517, index (row) #2=4 ("disabled index (row)"), index (col) #2=w517) -> (element #1=w495:dbl, element #2=w496:dbl)
                  n275 = Index Array(array=w492, index (row) #1=5 ("index (row)"), index (col) #1=w518, index (row) #2=4 ("disabled index (row)"), index (col) #2=w518) -> (element #1=w493:dbl, element #2=w494:dbl)
                  n276 = call "headingweightsum2.vi"("a"=0.5, "h2"=w509, "h1"=w497) -> ("a*h2+(1-a)*h1"=w498:dbl)  [unwired: 8 in]
                  n277 = call "rotm_siso.vi"("angle[rad]"=w509, "reverse"=TRUE, "y0"=w569, "x0"=w568, "y"=0.0, "x"=-10.0) -> ("y'"=w574:dbl, "x'"=w573:dbl)  [unwired: 4 in]
                  n278 = Multiply(x=w505, y=0.5) -> (x*y=w504:dbl)
                  n279 = Multiply(x=w533, y=0.5) -> (x*y=w535:dbl)
                  n280 = Multiply(x=w500, y=0.5) -> (x*y=w499:dbl)
                  n281 = Multiply(x=w538, y=0.5) -> (x*y=w536:dbl)
                  n282 = Build Array(w495, w496, w499, w536, w569, w574) -> (w564:dbl[])
                  n283 = Build Array(w493, w494, w504, w535, w568, w573) -> (w562:dbl[])
                  n284 = Build Array(w497, w497, w498, w509, w509, w509) -> (w566:dbl[])
                  n285 = Reverse 1D Array(array=w562) -> (reversed array=w563:dbl[])
                  n286 = Reverse 1D Array(array=w564) -> (reversed array=w565:dbl[])
                  n287 = Reverse 1D Array(array=w566) -> (reversed array=w567:dbl[])
                  n288 = Build Array(w563, w565, w567) -> (w559:dbl[][])
                  n289 = Transpose 2D Array(2D array=w559) -> (transposed array=w560:dbl[][])
                }
                frame True {
                  w592 = 1 ("disabled index (col)")
                  w593 = 0 ("disabled index (col)")
                  n290 = Index Array(array=w589, index (col) #1=1 ("disabled index (col)"), index (col) #2=0 ("index (col)")) -> (element #1=w633:dbl[], element #2=w628:dbl[])  [unwired: 2 in]
                  n291 = Multiply(x=0.5, y=w589) -> (x*y=w606:dbl[][])
                  n292 = global read "G_PATH.vi" "parking_point"() -> (w575:dbl[][])
                  n293 = global read "G_PATH.vi" "parking_point"() -> (w576:dbl[][])
                  n294 = global read "G_PATH.vi" "parking_point"() -> (w577:dbl[][])
                  n295 = Index Array(array=w606, index (col) #1=0 ("disabled index (col)"), index (col) #2=1 ("index (col)")) -> (element #1=w600:dbl[], element #2=w619:dbl[])  [unwired: 2 in]
                  n296 = Index Array(array=w633, index #1=0 ("index"), index #2=1 ("index")) -> (element #1=w625:dbl, element #2=w624:dbl)
                  n297 = Index Array(array=w628, index #1=0 ("index"), index #2=1 ("index")) -> (element #1=w623:dbl, element #2=w622:dbl)
                  n298 = Subtract(x=w625, y=w624) -> (x-y=w621:dbl)
                  n299 = Subtract(x=w623, y=w622) -> (x-y=w620:dbl)
                  n300 = Index Array(array=w600, index #1=3 ("index"), index #2=0 ("index")) -> (element #1=w588:dbl, element #2=w603:dbl, element #3=w604:dbl, element #4=w605:dbl)  [unwired: 2 in]
                  n301 = Index Array(array=w619, index #1=3 ("index"), index #2=0 ("index")) -> (element #1=w587:dbl, element #2=w616:dbl, element #3=w615:dbl, element #4=w614:dbl)  [unwired: 2 in]
                  n302 = Add(x=w588, y=w603) -> (x+y=w579:dbl)
                  n303 = Add(x=w604, y=w605) -> (x+y=w643:dbl)
                  n304 = Add(x=w587, y=w616) -> (x+y=w578:dbl)
                  n305 = Add(x=w615, y=w614) -> (x+y=w644:dbl)
                  n306 = Inverse Tangent (2 Input)(1:w620, 2:w621) -> (0:w586:dbl)
                  n307 = Index Array(array=w576, index (row)=4, index (col)=2 ("disabled index (col)")) -> (element=w584:dbl)
                  n308 = Add(x=w579, y=w643) -> (x+y=w608:dbl)
                  n309 = Add(x=w578, y=w644) -> (x+y=w613:dbl)
                  n310 = Index Array(array=w575, index (row) #1=5 ("index (row)"), index (col) #1=w592, index (row) #2=4 ("disabled index (row)"), index (col) #2=w592) -> (element #1=w582:dbl, element #2=w583:dbl)
                  n311 = Index Array(array=w577, index (row) #1=5 ("index (row)"), index (col) #1=w593, index (row) #2=4 ("disabled index (row)"), index (col) #2=w593) -> (element #1=w580:dbl, element #2=w581:dbl)
                  n312 = call "headingweightsum2.vi"("a"=0.5, "h2"=w586, "h1"=w584) -> ("a*h2+(1-a)*h1"=w585:dbl)  [unwired: 8 in]
                  n313 = call "rotm_siso.vi"("angle[rad]"=w586, "reverse"=TRUE, "y0"=w644, "x0"=w643, "y"=0.0, "x"=-10.0) -> ("y'"=w649:dbl, "x'"=w648:dbl)  [unwired: 4 in]
                  n314 = Multiply(x=w608, y=0.5) -> (x*y=w610:dbl)
                  n315 = Multiply(x=w613, y=0.5) -> (x*y=w611:dbl)
                  n316 = Build Array(w582, w583, w578, w611, w644, w649) -> (w639:dbl[])
                  n317 = Build Array(w580, w581, w579, w610, w643, w648) -> (w637:dbl[])
                  n318 = Build Array(w584, w584, w585, w586, w586, w586) -> (w641:dbl[])
                  n319 = Reverse 1D Array(array=w637) -> (reversed array=w638:dbl[])
                  n320 = Reverse 1D Array(array=w639) -> (reversed array=w640:dbl[])
                  n321 = Reverse 1D Array(array=w641) -> (reversed array=w642:dbl[])
                  n322 = Build Array(w638, w640, w642) -> (w634:dbl[][])
                  n323 = Transpose 2D Array(2D array=w634) -> (transposed array=w635:dbl[][])
                }
              }
              "parkingpoint" <- w489
            }
            frame #2 {
              n324 = global read "G_VEH.vi" "xparking"() -> (w674:T3)
              n325 = global read "G_VEH.vi" "xparking"() -> (w663:T3)
              n326 = Divide(x=15.0 ("y"), y=180.0) -> (x/y=w656:dbl)
              n327 = local read "parkingpoint"() -> (w676:dbl[][])
              n328 = Unbundle By Name(w674) -> ("x"=w672:dbl, "y"=w662:dbl)
              n329 = Unbundle By Name(w663) -> ("h"=w661:dbl)
              n330 = Index Array(array=w676, index (row)=2 ("index")) -> (element=w678:dbl[])  [unwired: 1 in]
              n331 = Multiply(x=w656, y=3.141592653589793) -> (x*y=w654:dbl)
              n332 = Index Array(array=w678, index #1=0 ("index")) -> (element #1=w673:dbl, element #2=w671:dbl, element #3=w650:dbl)  [unwired: 2 in]
              n333 = Subtract(x=w672, y=w673) -> (x-y=w669:dbl)
              n334 = Subtract(x=w662, y=w671) -> (x-y=w670:dbl)
              n335 = call "headingoperater.vi"("h1"=w661, "h2"=w650) -> ("h2-h1"=w660:dbl)  [unwired: 8 in, 1 out]
              n336 = Square(x=w669) -> (x^2=w668:dbl)
              n337 = Square(x=w670) -> (x^2=w667:dbl)
              n338 = Absolute Value(x=w660) -> (abs(x)=w659:dbl)
              n339 = Add(x=w668, y=w667) -> (x+y=w666:dbl)
              n340 = Less?(x=w659, y=w654) -> (x < y?=w652:bool)
              n341 = Square Root(x=w666) -> (sqrt(x)=w665:dbl)
              n342 = Less?(x=w665, y=1.3) -> (x < y?=w653:bool)
              n343 = And(x=w653, y=w652) -> (x .and. y?=w651:bool)
              n344 = case shown="True" w651 {
                frame False {
                }
                frame True {
                  n345 = global read "G_PATH.vi" "parking_point"() -> (w680:dbl[][])
                  n346 = local read "parkingpoint"() -> (w686:dbl[][])
                  n347 = stacked-sequence {
                    tunnel: w686 -> [w839 w850 w858]
                    tunnel: w680 -> [w836 w847 w855]
                    tunnel: [w830 _ _] -> w688
                    tunnel: [_ w841 _] -> w689
                    tunnel: [_ _ w852] -> w690
                    tunnel: "a" -> [w829 w840 w851]
                    frame #0 {
                      n348 = Decrement(x=w829) -> (x-1=w834:dbl)
                      n349 = Index Array(array=w839, index (col)=0 ("disabled index (col)")) -> (element=w835:dbl[])  [unwired: 1 in]
                      n350 = Index Array(array=w836, index (col)=0 ("disabled index (col)")) -> (element=w833:dbl[])  [unwired: 1 in]
                      n351 = Multiply(x=w835, y=w829) -> (x*y=w832:dbl[])
                      n352 = Multiply(x=w834, y=w833) -> (x*y=w831:dbl[])
                      n353 = Subtract(x=w832, y=w831) -> (x-y=w830:dbl[])
                    }
                    frame #1 {
                      n354 = Decrement(x=w840) -> (x-1=w845:dbl)
                      n355 = Index Array(array=w850, index (col)=1 ("disabled index (col)")) -> (element=w846:dbl[])  [unwired: 1 in]
                      n356 = Index Array(array=w847, index (col)=1 ("disabled index (col)")) -> (element=w844:dbl[])  [unwired: 1 in]
                      n357 = Multiply(x=w846, y=w840) -> (x*y=w843:dbl[])
                      n358 = Multiply(x=w845, y=w844) -> (x*y=w842:dbl[])
                      n359 = Subtract(x=w843, y=w842) -> (x-y=w841:dbl[])
                    }
                    frame #2 {
                      n360 = Index Array(array=w858, index (col)=2 ("disabled index (col)")) -> (element=w854:dbl[])  [unwired: 1 in]
                      n361 = Index Array(array=w855, index (col)=2 ("disabled index (col)")) -> (element=w853:dbl[])  [unwired: 1 in]
                      n362 = for {
                        tunnel: w854 -> [w861] mode=indexing
                        tunnel: w853 -> [w862] mode=indexing
                        tunnel: w851 -> [w860]
                        tunnel: [w859] -> w852 mode=indexing
                        n363 = call "headingweightsum2.vi"("a"=w860, "h2"=w861, "h1"=w862) -> ("a*h2+(1-a)*h1"=w859:dbl)  [unwired: 8 in]
                      }
                    }
                  }
                  n364 = Build Array(w688, w689, w690) -> (w687:dbl[][])
                  n365 = Transpose 2D Array(2D array=w687) -> (transposed array=w679:dbl[][])
                  n366 = Subtract(x=w686, y=w679) -> (x-y=w685:dbl[][])
                  n367 = global write "G_PATH.vi" "parking_point"(w679) -> ()
                  n368 = Absolute Value(x=w685) -> (abs(x)=w684:dbl[][])
                  n369 = Add Array Elements(numeric array=w684) -> (sum=w683:dbl)
                  n370 = Greater?(x=w683, y=1e-06) -> (0:w681:bool)
                  n371 = case shown="True" w681 {
                    frame False {
                    }
                    frame True {
                      n372 = flat-sequence {
                        frame #0 {
                          n373 = global read "G_PATH.vi" "parking_width"() -> (w694:dbl)
                          n374 = global read "G_PATH.vi" "parking_width"() -> (w693:dbl)
                          n375 = global read "G_PATH.vi" "parking_point"() -> (w695:dbl[][])
                          n376 = global read "G_VEH.vi" "parking_loop"() -> (w696:bool)
                          n377 = case shown="True" w696 {
                            tunnel: [0.5 ("y") 0.75 ("y")] -> w728
                            tunnel: [-0.5 ("y") -0.25 ("y")] -> w698
                            frame True {
                            }
                            frame False {
                            }
                          }
                          n378 = Index Array(array=w695, index (row)=1) -> (element=w715:dbl[])  [unwired: 1 in]
                          n379 = Index Array(array=w695, index (row)=3) -> (element=w731:dbl[])  [unwired: 1 in]
                          n380 = Multiply(x=w693, y=0.5) -> (x*y=w706:dbl)
                          n381 = Negate(x=w706) -> (-x=w719:dbl)
                          n382 = Index Array(array=w715, index #1=0 ("index")) -> (element #1=w716:dbl, element #2=w717:dbl, element #3=w707:dbl)  [unwired: 2 in]
                          n383 = Index Array(array=w731, index #1=0 ("index")) -> (element #1=w730:dbl, element #2=w729:dbl)  [unwired: 2 in, 1 out]
                          n384 = Build Array(w719, w706) -> (w720:dbl[])
                          n385 = Multiply(x=w694, y=w728) -> (x*y=w699:dbl)
                          n386 = Multiply(x=w694, y=w698) -> (x*y=w697:dbl)
                          n387 = Multiply(x=0.0 ("y"), y=w720) -> (x*y=w721:dbl[])
                          n388 = Build Array(w699, w697) -> (w727:dbl[])
                          n389 = call "rotm_mimo.vi"("angle[rad]"=w707, "reverse"=TRUE, "y0"=w717, "x0"=w716, "y"=w720, "x"=w721) -> ("Y"=w711:dbl[], "X"=w712:dbl[])  [unwired: 2 in, 2 out]
                          n390 = Multiply(x=0.0 ("y"), y=w727) -> (x*y=w726:dbl[])
                          n391 = call "rotm_mimo.vi"("angle[rad]"=w707, "reverse"=TRUE, "y0"=w729, "x0"=w730, "y"=w727, "x"=w726) -> ("Y"=w701:dbl[], "X"=w705:dbl[])  [unwired: 2 in, 2 out]
                          n392 = Index Array(array=w705, index=0) -> (element=w703:dbl)
                          n393 = Index Array(array=w701, index=0) -> (element=w700:dbl)
                          n394 = Build Array (concatenate)(w705, w712, w703) -> (w710:dbl[])
                          n395 = Build Array (concatenate)(w701, w711, w700) -> (w709:dbl[])
                          n396 = Build Array(w710, w709) -> (w708:dbl[][])
                          n397 = Transpose 2D Array(2D array=w708) -> (transposed array=w692:dbl[][])
                          n398 = global write "G_PATH.vi" "wpt_park"(w692) -> ()
                        }
                        frame #1 {
                          n399 = global read "G_VEH.vi" "xparking"() -> (w748:T3)
                          n400 = global read "G_PATH.vi" "parking_point"() -> (w738:dbl[][])
                          n401 = Array Size(array=w738) -> (size(s)=w739:i32[])
                          n402 = Index Array(array=w738, index (row)=2 ("index")) -> (element=w747:dbl[])  [unwired: 1 in]
                          n403 = Index Array(array=w747, index #1=0 ("index")) -> (element #1=w750:dbl, element #2=w751:dbl, element #3=w752:dbl)  [unwired: 2 in]
                          n404 = Index Array(array=w739, index=0) -> (element=w741:i32)
                          n405 = Decrement(x=w741) -> (x-1=w742:i32)
                          n406 = Bundle By Name(cluster=w748, "idx"=2 ("c_idx"), "x"=w750, "y"=w751, "h"=w752) -> (w753:T3)
                          n407 = for {
                            N: w742 -> [_]
                            tunnel: [w766] -> w743 mode=indexing
                            i -> [w774]
                            w780 = 2 ("disabled index (col)")
                            n408 = global read "G_PATH.vi" "parking_point"() -> (w754:dbl[][])
                            n409 = Increment(x=w774) -> (x+1=w781:i32)
                            n410 = Index Array(array=w754, index (row) #1=w774, index (row) #2=w781, index (row) #3=w774, index (row) #4=w781, index (col) #4=w780, index (row) #5=w774, index (col) #5=w780) -> (element #1=w773:dbl[], element #2=w764:dbl[], element #3=w760:dbl[], element #4=w779:dbl, element #5=w778:dbl)  [unwired: 3 in]
                            n411 = call "headingoperater.vi"("h1"=w778, "h2"=w779) -> ("h2-h1"=w777:dbl)  [unwired: 8 in, 1 out]
                            n412 = Index Array(array=w773, index #1=0 ("index")) -> (element #1=w771:dbl, element #2=w770:dbl, element #3=w769:dbl)  [unwired: 2 in]
                            n413 = Index Array(array=w764, index #1=0 ("index")) -> (element #1=w763:dbl, element #2=w762:dbl)  [unwired: 1 in]
                            n414 = Index Array(array=w760, index #1=0 ("index")) -> (element #1=w759:dbl, element #2=w755:dbl, element #3=w756:dbl)  [unwired: 2 in]
                            n415 = call "rotm_siso.vi"("angle[rad]"=w756, "y0"=w755, "x0"=w759, "y"=w762, "x"=w763) -> ("y'"=w757:dbl, "x'"=w758:dbl)  [unwired: 5 in]
                            n416 = call "cubic.vi"("h"=w777, "y"=w757, "x"=w758) -> ("b"=w775:dbl, "a"=w776:dbl)  [unwired: 5 in, 2 out]
                            n417 = Build Array(w771, w770, w769, w758, w776, w775, -5.0 ("element"), 0.0 ("element")) -> (w766:dbl[])
                          }
                          n418 = global write "G_VEH.vi" "xparking"(w753) -> ()
                          n419 = Transpose 2D Array(2D array=w743) -> (transposed array=w744:dbl[][])
                          n420 = global write "G_PATH.vi" "path_rev"(w744) -> ()
                        }
                        frame #2 {
                          n421 = global read "G_PATH.vi" "path_rev"() -> (w782:dbl[][])
                          n422 = global write "G_PATH.vi" "path"(w782) -> ()
                          n423 = global write "G_PATH.vi" "path_origin"(w782) -> ()
                        }
                        frame #3 {
                          w787 = dbl[] []
                          n424 = global read "G_PATH.vi" "path"() -> (w783:dbl[][])
                          n425 = Array Size(array=w783) -> (size(s)=w786:i32[])
                          n426 = Index Array(array=w786, index=1) -> (element=w784:i32)
                          n427 = for {
                            N: w784 -> [_]
                            shift-right: [w795] -> w788
                            shift-left: w787 -> [w797]
                            shift-right: [w792] -> w789
                            shift-left: w787 -> [w794]
                            tunnel: w783 -> [w790]
                            i -> [w791]
                            n428 = Index Array(array=w790, index (col)=w791) -> (element=w811:dbl[])  [unwired: 1 in]
                            n429 = global read "G_VEH.vi" "path_size_div"() -> (w806:dbl)
                            n430 = Index Array(array=w811, index #1=3 ("index"), index #4=0 ("index")) -> (element #1=w805:dbl, element #2=w808:dbl, element #3=w807:dbl, element #4=w800:dbl, element #5=w799:dbl, element #6=w798:dbl)  [unwired: 4 in]
                            n431 = Less?(x=w806, y=w805) -> (x < y?=w809:bool)
                            n432 = case shown="True" w809 {
                              tunnel: w805 -> [_ w827]
                              tunnel: w808 -> [_ w822]
                              tunnel: w807 -> [_ w821]
                              tunnel: [w812 w817] -> w804
                              tunnel: [w812 w816] -> w803
                              frame False {
                                w812 = dbl[] [0.0]
                              }
                              frame True {
                                n433 = global read "G_VEH.vi" "path_size_div"() -> (w823:dbl)
                                n434 = Divide(x=w827, y=w823) -> (x/y=w826:dbl)
                                n435 = Round Toward -Infinity(1:w826) -> (0:w825:dbl)
                                n436 = To Long Integer(number=w825) -> (32bit integer=w814:i32)
                                n437 = Max & Min(x=w814, y=5000) -> (min(x,y)=w813:i32)  [unwired: 1 out]
                                n438 = for {
                                N: w813 -> [_]
                                tunnel: [w828] -> w824 mode=indexing
                                i -> [w828]
                                }
                                n439 = Multiply(x=w824, y=w823) -> (x*y=w817:dbl[])
                                n440 = Square(x=w817) -> (x^2=w818:dbl[])
                                n441 = Compound Arithmetic op=MULTIPLY(w817, w818, w822) -> (w820:dbl[])
                                n442 = Compound Arithmetic op=MULTIPLY(w818, w821) -> (w819:dbl[])
                                n443 = Add(x=w820, y=w819) -> (x+y=w816:dbl[])
                              }
                            }
                            n444 = call "rotm_mimo.vi"("angle[rad]"=w798, "reverse"=TRUE, "y0"=w799, "x0"=w800, "y"=w803, "x"=w804) -> ("Y"=w793:dbl[], "X"=w796:dbl[])  [unwired: 2 in, 2 out]
                            n445 = Build Array (concatenate)(w794, w793) -> (w792:dbl[])
                            n446 = Build Array (concatenate)(w797, w796) -> (w795:dbl[])
                          }
                          n447 = global write "G_PATH.vi" "y origin"(w789) -> ()
                          n448 = global write "G_PATH.vi" "x origin"(w788) -> ()
                        }
                      }
                    }
                  }
                }
              }
            }
          }
        }
        frame True {
        }
      }
    }
    frame #4 {
      n449 = local read "M6006"() -> (w869:T1)
      n450 = Tick Count (ms)() -> (millisecond timer value=w876:u32)
      n451 = local read "tic"() -> (w874:u32)
      n452 = Unbundle By Name(w869) -> ("lcc[1]"=w871:sgl, "lcc[0]"=w872:sgl, "attitude[2]"=w870:sgl)
      n453 = global read "G_PATH.vi" "wpt_park"() -> (w863:dbl[][])
      n454 = Subtract(x=w876, y=w874) -> (x-y=→"time":u32)
      n455 = Negate(x=w870) -> (-x=w873:sgl)
      n456 = Index Array(array=w863, index (col) #1=0 ("disabled index (col)")) -> (element #1=w867:dbl[], element #2=w868:dbl[])  [unwired: 3 in]
      n457 = call "rotm_mimo.vi"("angle[rad]"=w873, "y0"=w872, "x0"=w871, "y"=w868, "x"=w867) -> ("Y"=w864:dbl[], "X"=w865:dbl[])  [unwired: 3 in, 2 out]
    }
    frame #5 {
      n458 = flat-sequence {
        tunnel: [w924] -> w880
        tunnel: w878 -> [w905]
        frame #0 {
          n459 = local read "lane"() -> (w915:dbl[][])
          n460 = local read "box"() -> (w910:dbl[][])
          n461 = local read "obs"() -> (w923:dbl[][])
          n462 = call "Convert to Dynamic Data6"("Array"=w905) -> ("Dynamic Data Type"=w911:dynamicdata)  [unwired: 3 in]
          n463 = local read "sensor_lane"() -> (w907:dbl[][])
          n464 = local read "sensor_obs"() -> (w906:dbl[][])
          n465 = Index Array(array=w910, index (col)=0 ("disabled index (col)")) -> (element=w908:dbl[])  [unwired: 1 in]
          n466 = Index Array(array=w915, index (col)=0 ("disabled index (col)")) -> (element=w916:dbl[])  [unwired: 1 in]
          n467 = Index Array(array=w923, index (col)=0 ("disabled index (col)")) -> (element=w922:dbl[])  [unwired: 1 in]
          n468 = call "Convert to Dynamic Data5"("Array"=w908) -> ("Dynamic Data Type"=w912:dynamicdata)  [unwired: 3 in]
          n469 = call "Convert to Dynamic Data4"("Array"=w916) -> ("Dynamic Data Type"=w914:dynamicdata)  [unwired: 3 in]
          n470 = call "Convert to Dynamic Data2"("Array"=w922) -> ("Dynamic Data Type"=w921:dynamicdata)  [unwired: 3 in]
          n471 = Index Array(array=w907, index (col)=0 ("disabled index (col)")) -> (element=w919:dbl[])  [unwired: 1 in]
          n472 = Index Array(array=w906, index (col)=0 ("disabled index (col)")) -> (element=w926:dbl[])  [unwired: 1 in]
          n473 = call "Convert to Dynamic Data3"("Array"=w919) -> ("Dynamic Data Type"=w913:dynamicdata)  [unwired: 3 in]
          n474 = call "Convert to Dynamic Data"("Array"=w926) -> ("Dynamic Data Type"=w925:dynamicdata)  [unwired: 3 in]
          n475 = Merge Signals(w914, w913, w921, w925, w912, w911) -> (w924:dynamicdata)
        }
      }
      n476 = flat-sequence {
        tunnel: [w901] -> w879
        tunnel: w877 -> [w882]
        frame #0 {
          n477 = local read "lane"() -> (w892:dbl[][])
          n478 = local read "box"() -> (w887:dbl[][])
          n479 = local read "obs"() -> (w900:dbl[][])
          n480 = call "Convert to Dynamic Data12"("Array"=w882) -> ("Dynamic Data Type"=w888:dynamicdata)  [unwired: 3 in]
          n481 = local read "sensor_lane"() -> (w884:dbl[][])
          n482 = local read "sensor_obs"() -> (w883:dbl[][])
          n483 = Index Array(array=w887, index (col)=1 ("disabled index (col)")) -> (element=w885:dbl[])  [unwired: 1 in]
          n484 = Index Array(array=w892, index (col)=1 ("disabled index (col)")) -> (element=w893:dbl[])  [unwired: 1 in]
          n485 = Index Array(array=w900, index (col)=1 ("disabled index (col)")) -> (element=w899:dbl[])  [unwired: 1 in]
          n486 = call "Convert to Dynamic Data11"("Array"=w885) -> ("Dynamic Data Type"=w889:dynamicdata)  [unwired: 3 in]
          n487 = call "Convert to Dynamic Data10"("Array"=w893) -> ("Dynamic Data Type"=w891:dynamicdata)  [unwired: 3 in]
          n488 = call "Convert to Dynamic Data8"("Array"=w899) -> ("Dynamic Data Type"=w898:dynamicdata)  [unwired: 3 in]
          n489 = Index Array(array=w884, index (col)=1 ("disabled index (col)")) -> (element=w896:dbl[])  [unwired: 1 in]
          n490 = Index Array(array=w883, index (col)=1 ("disabled index (col)")) -> (element=w903:dbl[])  [unwired: 1 in]
          n491 = call "Convert to Dynamic Data9"("Array"=w896) -> ("Dynamic Data Type"=w890:dynamicdata)  [unwired: 3 in]
          n492 = call "Convert to Dynamic Data7"("Array"=w903) -> ("Dynamic Data Type"=w902:dynamicdata)  [unwired: 3 in]
          n493 = Merge Signals(w891, w890, w898, w902, w889, w888) -> (w901:dynamicdata)
        }
      }
      n494 = call "Build XY Graph"("Y Input"=w879, "X Input"=w880) -> ("XY Graph"=→"XY Graph":cluster{"Y":dbl[], "Y":dbl[]}[])  [unwired: 3 in, 6 out]
    }
  }
